vi "Destroy.vi"(8 "ErrorIn":errorcluster, 11 "ObjectIn":refnum<class "YAFTAF.lvclass">) -> (0 "ErrorOut":errorcluster, 3 "ObjectOut":refnum<class "YAFTAF.lvclass">)   [LabVIEW 2021, in "YAFTAF.lvclass"]
uses:
  YAFTAF.lvclass
  C:/Localdata/Projects/TriekselSoft/TriekselsoftApplicationFramework/Source/.Externals/Library_YAF/YActor/YActor.lvclass
  YActor/YActor.lvclass/YActor.ctl
  YActor/ExeCmd_sync.vi
  YActor/private/SendCommand.vi
  YActor/private/WaitForReply.vi
  YActor/private/CreateLocalVI.vi
  YActor/private/ExeuteInlineVI.vi
  YActor/private/GetRemoteVIRef.vi
  YActor/private/GetNameOfVI.vi
  YActor/QuickCast.vi
  YAFTAF_Destructor.vi
  YActor/private/VINameProperty.vi
  YActor/private/MessageCounter.vi
  YActor/InlineReferencePool.vi
  YActor/private/ExecuteVI.vi
  YActor/YActor.lvclass
  YAFTAF.lvclass/YAFTAF.ctl
  C:/Localdata/Projects/TriekselSoft/TriekselsoftApplicationFramework/Source/.Externals/Interface_UserInterface_IFrontPanel/IFrontPanel/IFrontPanel.lvclass
  C:/Localdata/Projects/TriekselSoft/TriekselsoftApplicationFramework/Source/IInterface/IInterface.lvclass
  C:/Localdata/Projects/TriekselSoft/TriekselsoftApplicationFramework/Source/.Externals/Interface_Object_ICreateDestroy/ICreateDestroy/ICreateDestroy.lvclass
  C:/Localdata/Projects/TriekselSoft/TriekselsoftApplicationFramework/Source/.Externals/Interface_Object_IPersistentData/IPersistentData/IPersistentData.lvclass
  C:/Localdata/Projects/TriekselSoft/TriekselsoftApplicationFramework/Source/.Externals/Interface_TAF_ITAFObject/ITAFObject/ITAFObject.lvclass
  C:/Localdata/Projects/TriekselSoft/TriekselsoftApplicationFramework/Source/.Externals/Library_YAF/YAFTAF/YAFTAF.lvclass
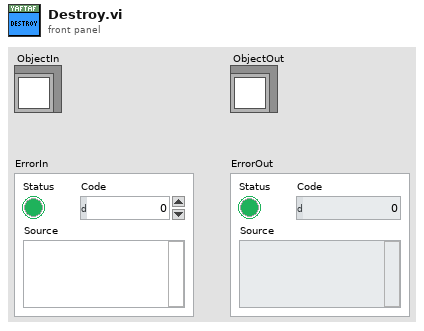
[diagram p1: front panel]
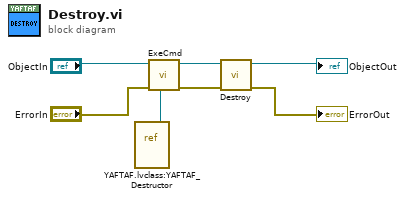
[diagram p0: block diagram]
diagram:
  n1 = vi-ref "YAFTAF.lvclass:YAFTAF_Destructor.vi"() -> (w3:refnum<vi>)
  n2 = call-poly "ExeCmd.vi"("CmdVIRef"=w3, "ErrorIn"="ErrorIn", "YActorIn"="ObjectIn") -> ("ErrorOut"=w6:errorcluster, "YActorOut"=w2:refnum<class "YAFTAF.lvclass">)  [unwired: 6 in, 1 out]
  n3 = call-parent "Destroy.vi"("ErrorIn"=w6, "YActorIn"=w2) -> ("ErrorOut"=→"ErrorOut":errorcluster, "YActorOut"=→"ObjectOut":refnum<class "YAFTAF.lvclass">)  [unwired: 8 in]
